vi "Programmatically Invert Roi.vi"(10 "Invert Roi":bool[](array[boolean]), 11 "Table Roi In":i32[][](array[numeric])) -> (3 "Table Roi Out":i32[][](array[numeric]))   [LabVIEW 2023]
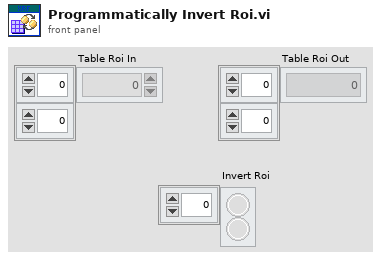
[diagram p1: front panel]
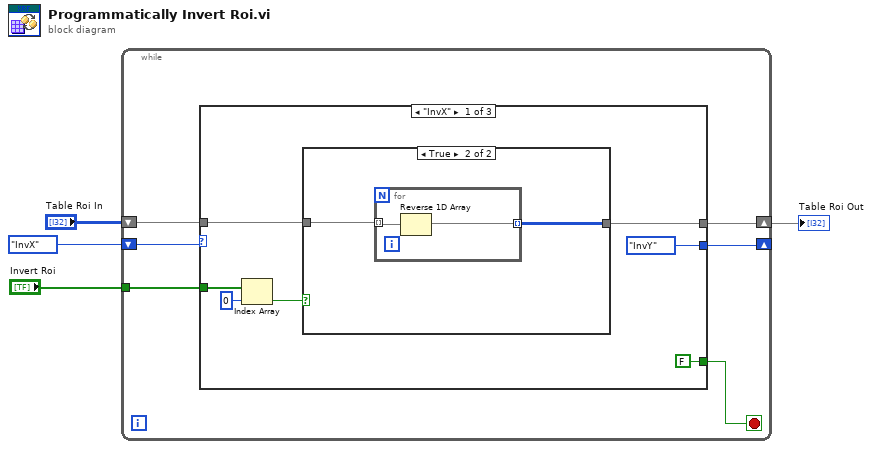
[diagram p0: block diagram]
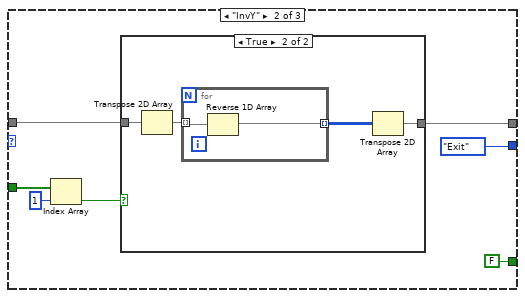
[diagram p3: hidden frame]
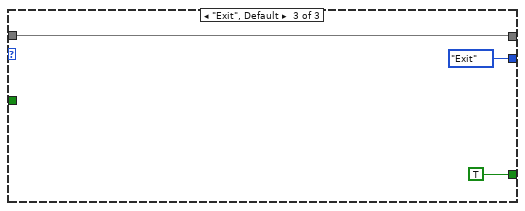
[diagram p5: hidden frame]
diagram:
  n1 = while {
    shift-right: [w8] -> _
    shift-left: enum16{"InvX", "InvY", "Exit"}."InvX" -> [w10]
    tunnel: "Invert Roi" -> [w7]
    shift-right: [w5] -> w1
    shift-left: "Table Roi In" -> [w6]
    stop <- w9 stop-if-true
    n2 = case shown="\"InvX\"" w10 {
      tunnel: [FALSE FALSE TRUE] -> w9
      tunnel: [enum16{"InvX", "InvY", "Exit"}."InvY" enum16{"InvX", "InvY", "Exit"}."Exit" enum16{"InvX", "InvY", "Exit"}."Exit"] -> w8
      tunnel: w7 -> [w15 w26 _]
      tunnel: w6 -> [w13 w25 w37]
      tunnel: [w11 w24 w37] -> w5
      frame "InvX" {
        n3 = Index Array(array=w15, index=0) -> (element=w12:bool)
        n4 = case shown="True" w12 {
          tunnel: w13 -> [w18 w20]
          tunnel: [w18 w19] -> w11
          frame False {
          }
          frame True {
            n5 = for {
              tunnel: w20 -> [w22] mode=indexing
              tunnel: [w21] -> w19 mode=indexing
              n6 = Reverse 1D Array(array=w22) -> (reversed array=w21:i32[])
            }
          }
        }
      }
      frame "InvY" {
        n7 = Index Array(array=w26, index=1) -> (element=w23:bool)
        n8 = case shown="True" w23 {
          tunnel: w25 -> [w30 w32]
          tunnel: [w30 w31] -> w24
          frame False {
          }
          frame True {
            n9 = Transpose 2D Array(2D array=w32) -> (transposed array=w33:i32[][])
            n10 = for {
              tunnel: w33 -> [w36] mode=indexing
              tunnel: [w35] -> w34 mode=indexing
              n11 = Reverse 1D Array(array=w36) -> (reversed array=w35:i32[])
            }
            n12 = Transpose 2D Array(2D array=w34) -> (transposed array=w31:i32[][])
          }
        }
      }
      frame "Exit", Default {
      }
    }
  }
  "Table Roi Out" <- w1
